vi "Calc - DCF.vi"(7 "WBMeas":dbl format="%0.2f", 10 "DeltaB":dbl format="%0.2f", 11 "ThetaB":dbl format="%0.2f") -> (3 "DCF":dbl format="%0.2f")   [LabVIEW 2018, in "Controller (Host).lvlib"]
uses:
  Controller (Host).lvlib
  <vilib>/ptbypt/NI_PtbyPt.lvlib
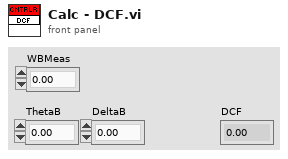
[diagram p1: front panel]
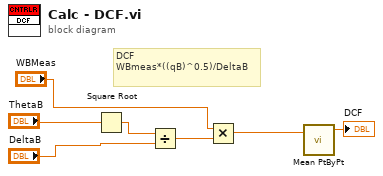
[diagram p0: block diagram]
diagram:
  # "DCF \nWBmeas*((qB)^0.5)/DeltaB"
  n1 = Square Root(x="ThetaB") -> (sqrt(x)=w6:dbl)
  n2 = Divide(x=w6, y="DeltaB") -> (x/y=w7:dbl)
  n3 = Multiply(x="WBMeas", y=w7) -> (x*y=w5:dbl)
  n4 = call <vilib>:"Mean PtByPt.vi"("x"=w5) -> ("mean"=→"DCF":dbl)  [unwired: 3 in, 1 out]
